vi "Laser power on,off (simple).vi"(2 "Blue Laser on":bool, 3 "Green Laser on":bool) -> (0 "Blue laser setting error":errorcluster, 1 "Green laser setting error":errorcluster)   [LabVIEW 2014]
uses:
  Laser enum.ctl
  Commands.ctl
panel:
  # "PN 04/11/2014"
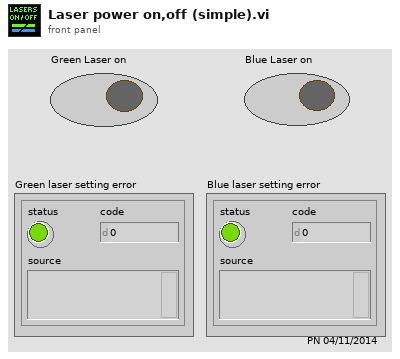
[diagram p1: front panel]
types:
  T1 = typedef "Commands.ctl" = u8
  T2 = typedef "Laser enum.ctl" = u8
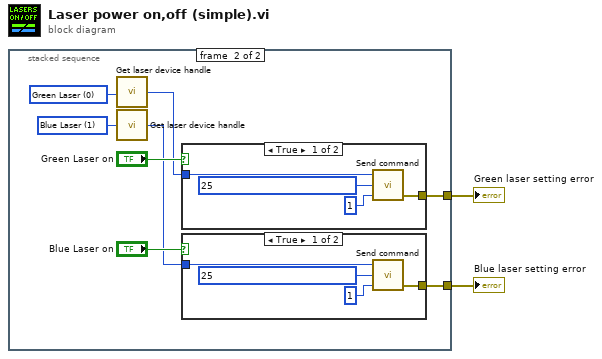
[diagram p0: block diagram]
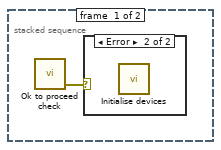
[diagram p2: hidden frame]
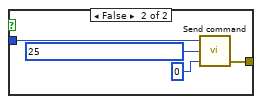
[diagram p4: hidden frame]
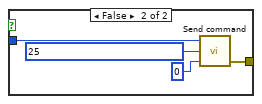
[diagram p5: hidden frame]
diagram:
  n1 = stacked-sequence {
    tunnel: [_ w10] -> w2
    tunnel: [_ w8] -> w1
    frame #0 {
      n2 = call "Ok to proceed check.vi"() -> ("Ok to proceed (error)"=w3:errorcluster)  [unwired: 3 in, 2 out]
      n3 = case shown="Error" w3 {
        frame No Error {
        }
        frame Error {
          n4 = call "Initialise devices.vi"() -> ()  [unwired: 6 in, 5 out]
        }
      }
    }
    frame #1 {
      w4 = T2 1 items=["Green Laser", "Blue Laser"] ("Selected laser")
      w5 = T2 0 items=["Green Laser", "Blue Laser"] ("Selected laser")
      n5 = call "Get laser device handle.vi"("Selected laser"=w5) -> ("Device handle"=w7:u32)
      n6 = call "Get laser device handle.vi"("Selected laser"=w4) -> ("Device handle"=w6:u32)
      n7 = case shown="True" "Green Laser on" {
        tunnel: w7 -> [w23 w27]
        tunnel: [w21 w25] -> w10
        frame True {
          n8 = call "Send command.vi"("Value"=u16 1, "Command"=T1 25, "Device handle"=w23) -> ("Error"=w21:errorcluster)  [unwired: 2 out]
        }
        frame False {
          n9 = call "Send command.vi"("Value"=u16 0, "Command"=T1 25, "Device handle"=w27) -> ("Error"=w25:errorcluster)  [unwired: 2 out]
        }
      }
      n10 = case shown="True" "Blue Laser on" {
        tunnel: w6 -> [w15 w19]
        tunnel: [w13 w17] -> w8
        frame True {
          n11 = call "Send command.vi"("Value"=u16 1, "Command"=T1 25, "Device handle"=w15) -> ("Error"=w13:errorcluster)  [unwired: 2 out]
        }
        frame False {
          n12 = call "Send command.vi"("Value"=u16 0, "Command"=T1 25, "Device handle"=w19) -> ("Error"=w17:errorcluster)  [unwired: 2 out]
        }
      }
    }
  }
  "Green laser setting error" <- w2
  "Blue laser setting error" <- w1
